vi "Test Base64 Encoder and Decoder.vi"() -> ()   [LabVIEW 2019]
uses:
  source-base64/OpenSerializer.base64.lvlib
panel:
  out "Variant 4":variant
  out "invalid type":errorcluster
  out "error out":errorcluster
  out "Variant 2":variant
  out "Variant":variant
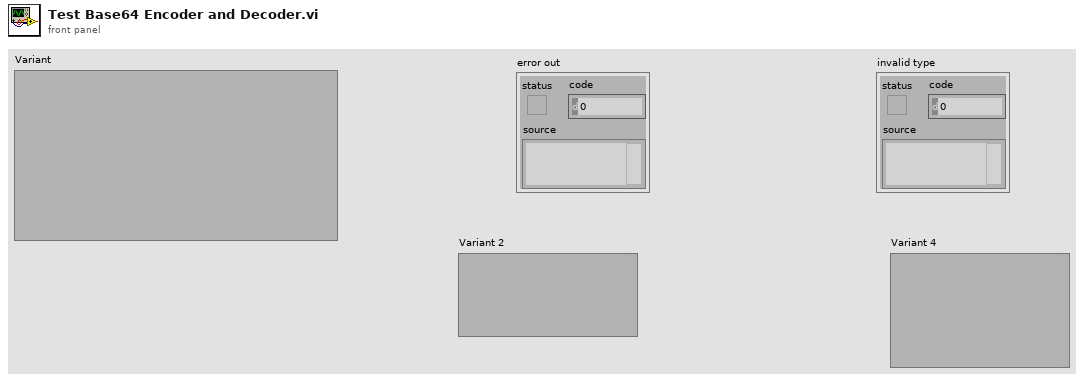
[diagram p1: front panel]
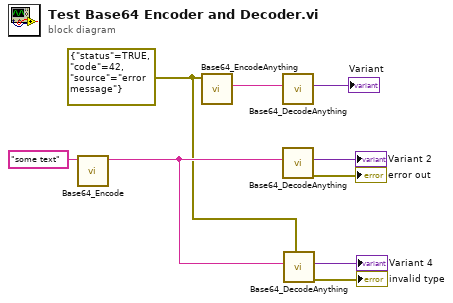
[diagram p0: block diagram]
diagram:
  w1 = errorcluster {"status"=TRUE, "code"=42, "source"="error message"} ("error constant")
  n1 = call "Base64_Encode.vi"("String"="some text") -> ("Encoded String"=w2:string)  [unwired: 9 in, 1 out]
  n2 = call "Base64_EncodeAnything.vi"("Variant"=w1) -> ("Encoded Payload"=w8:string)  [unwired: 8 in, 2 out]
  n3 = call "Base64_DecodeAnything.vi"("Encoded Payload"=w8) -> ("Variant"=→"Variant":variant)  [unwired: 9 in, 1 out]
  n4 = call "Base64_DecodeAnything.vi"("Encoded Payload"=w2) -> ("error out"=→"error out":errorcluster, "Variant"=→"Variant 2":variant)  [unwired: 9 in]
  n5 = call "Base64_DecodeAnything.vi"("Type (Adapt)"=w1, "Encoded Payload"=w2) -> ("error out"=→"invalid type":errorcluster, "Variant"=→"Variant 4":variant)  [unwired: 8 in]
